vi "initialise.vi"(8 "error in (no error)":errorcluster, 11 "NetworkWinX32 in":refnum<class "NetworkWinX32.lvclass">) -> (0 "error out":errorcluster, 3 "NetworkWinX32 out":refnum<class "NetworkWinX32.lvclass">)   [LabVIEW 2011, in "Hardware.lvlib" / "HWControllers.lvlib" / "NetworkWinX32.lvclass"]
uses:
  NetworkWinX32.lvclass
  NetworkWinX32.lvclass/NetworkWinX32.ctl
  Channels/Camera/WinX32_SA/WinX32Camera.lvclass
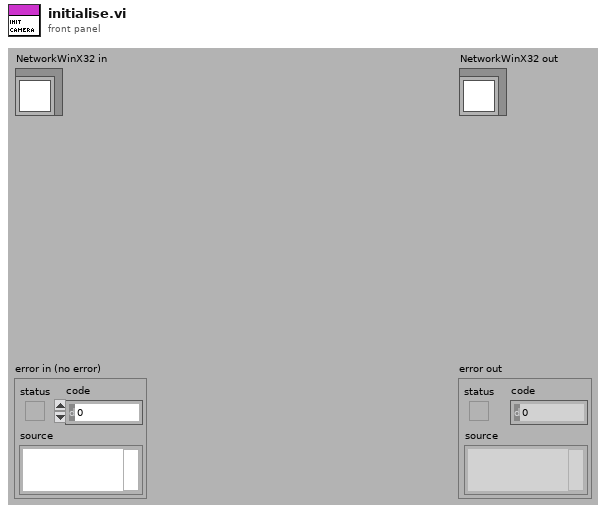
[diagram p1: front panel]
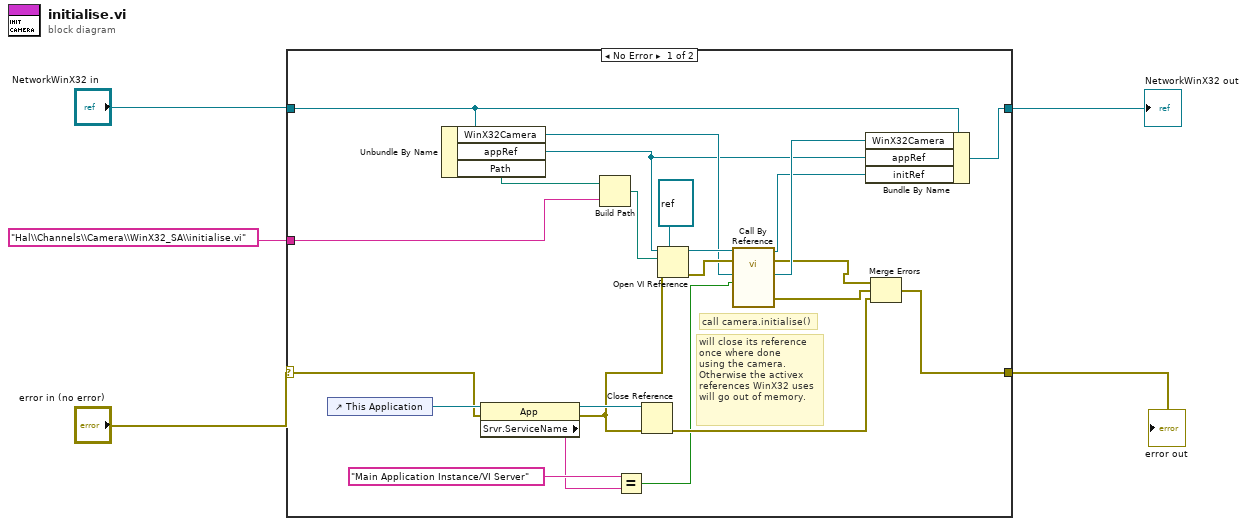
[diagram p0: block diagram]
diagram:
  n1 = case shown="No Error" "error in (no error)" {
    selector: "error in (no error)" -> [w11 w30]
    tunnel: [w17 w30] -> w3
    tunnel: [w16 w29] -> w4
    tunnel: "NetworkWinX32 in" -> [w21 w29]
    tunnel: "Hal\\Channels\\Camera\\WinX32_SA\\initialise.vi" ("viPath") -> [w27 _]
    frame No Error {
      # "will close its reference\nonce where done\nusing the camera.\nOtherwise the activex\nreferences WinX32 uses\nwill go out of memory."
      # "call camera.initialise()"
      n2 = control-ref of="This Application"() -> (w15:refnum<vi>)
      n3 = Unbundle By Name(w21) -> ("WinX32Camera"=w22:refnum<class "WinX32Camera.lvclass">, "appRef"=w19:refnum<vi>, "Path"=w26:path)
      n4 = property class="App"(reference=w15, error in=w11) -> (reference out=w14:refnum<vi>, error out=w10:errorcluster, "Srvr.ServiceName"=w12:string)
      n5 = Build Path(base path=w26, name or relative path=w27) -> (appended path=w28:path)
      n6 = Equal?(x="Main Application Instance/VI Server", y=w12) -> (x = y?=w8:bool)
      n7 = Close Reference(reference=w14, error in (no error)=w10) -> (error out=w9:errorcluster)
      n8 = Open VI Reference(type specifier VI Refnum (for type only)=refnum<vi> refnum, application reference (local)=w19, vi path=w28, error in (no error)=w10) -> (vi reference=w24:refnum<vi>, error out=w23:errorcluster)  [unwired: 2 in]
      n9 = call-by-ref "?"(reference=w24, error in=w23, "main_app_instance"=w8, "WinX32Camera in"=w22) -> (reference out=w6:refnum<vi>, error out=w7:errorcluster, 0:"error out"=w18:errorcluster, "WinX32Camera out"=w20:refnum<class "WinX32Camera.lvclass">)  [unwired: 8 in]
      n10 = Bundle By Name(cluster=w21, "WinX32Camera"=w20, "appRef"=w19, "initRef"=w6) -> (w16:refnum<class "NetworkWinX32.lvclass">)
      n11 = Merge Errors(w7, w18, w9) -> (w17:errorcluster)
    }
    frame Error {
    }
  }
  "error out" <- w3
  "NetworkWinX32 out" <- w4
